vi "Test Report is Opened on Test Start.vi"(8 "error in (no error)":errorcluster, 11 "XML Report Test in":refnum<class "Report Generator Test.lvclass">) -> (0 "error out":errorcluster, 3 "XML Report Test out":refnum<class "Report Generator Test.lvclass">)   [LabVIEW 2020, in "Report Generator Test.lvclass"]
uses:
  Report Generator Test.lvclass
  C:/Program Files (x86)/National Instruments/LabVIEW 2020/vi.lib/Astemes/LUnit/Test Case.lvclass
  <vilib>/Astemes/LUnit/Test Case.lvclass/Test Case.ctl
  <vilib>/Astemes/LUnit/Set Assertion Type.vi
  <vilib>/Astemes/LUnit/Palette/Pass.vi
  <vilib>/Astemes/LUnit/Palette/Fail.vi
  <vilib>/Astemes/LUnit/Add test result.vi
  <vilib>/Astemes/LUnit/LUnit Record Assertion Result.vi
  <vilib>/Astemes/LUnit/LUnit Aggregate Assertion Results.vi
  <vilib>/Astemes/LUnit/Method Result/LUnit Merge Status.vi
  <vilib>/Astemes/LUnit/LUnit Concatenate result strings.vi
  Test Doubles/Mock Report/Mock Report.lvclass
  <vilib>/Astemes/LUnit/Test Case.lvclass
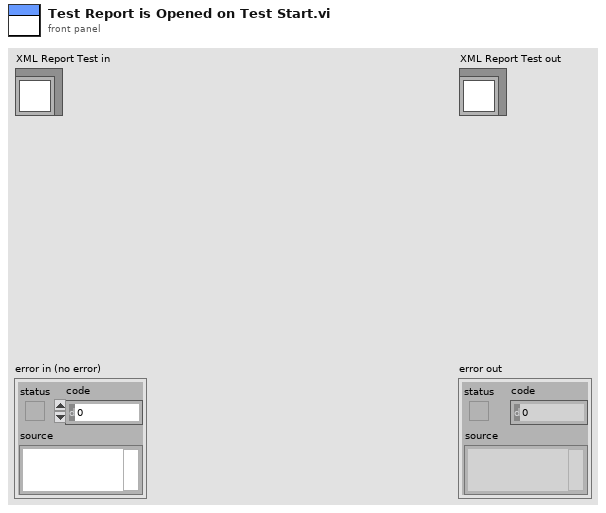
[diagram p1: front panel]
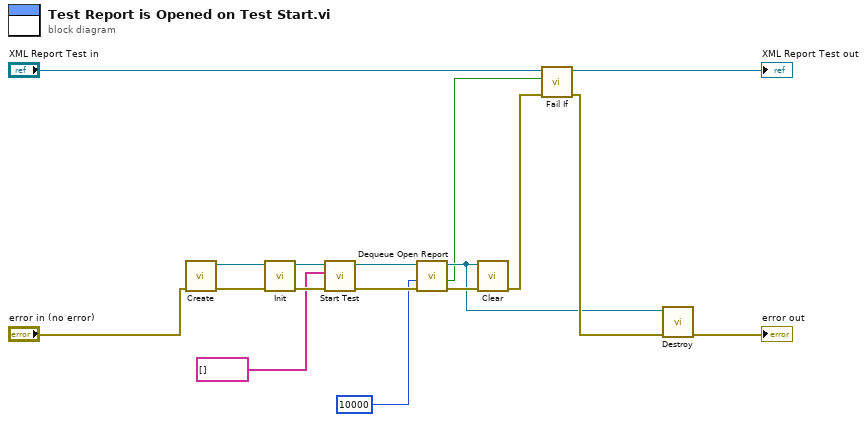
[diagram p0: block diagram]
diagram:
  n1 = call "Create.vi"("error in (no error)"="error in (no error)") -> ("error out"=w6:errorcluster, "Mock Report out"=w8:refnum<class "Mock Report.lvclass">)  [unwired: 9 in]
  n2 = call-dynamic "Init.vi"("error in (no error)"=w6, "XML Report in"=w8) -> ("error out"=w13:errorcluster, "XML Report out"=w14:refnum<class "Mock Report.lvclass">)  [unwired: 8 in]
  n3 = call-dynamic "Start Test.vi"("error in (no error)"=w13, "Tests"=string[] [], "XML Report in"=w14) -> ("error out"=w12:errorcluster, "XML Report out"=w11:refnum<class "Mock Report.lvclass">)  [unwired: 7 in]
  n4 = call "Dequeue Open Report.vi"("error in (no error)"=w12, "timeout in ms (0)"=10000, "Mock Report in"=w11) -> ("error out"=w10:errorcluster, "timed out?"=w1:bool, "Mock Report out"=w4:refnum<class "Mock Report.lvclass">)  [unwired: 5 in, 1 out]
  n5 = call-dynamic "Clear.vi"("error in (no error)"=w10, "XML Report in"=w4) -> ("error out"=w9:errorcluster)  [unwired: 9 in]
  n6 = call <vilib>:"Fail If.vi"("error in (no error)"=w9, "Fail?"=w1, "LUnit Test Case In"="XML Report Test in") -> ("error out"=w15:errorcluster, "LUnit Test Case Out"=→"XML Report Test out":refnum<class "Report Generator Test.lvclass">)  [unwired: 7 in]
  n7 = call "Destroy.vi"("error in (no error)"=w15, "Mock Report in"=w4) -> ("error out"=→"error out":errorcluster)  [unwired: 9 in]
